vi "UNIX_date.vi"(8 "error in (no error)":errorcluster) -> (0 "error out":errorcluster, 3 "current time":timestamp)   [LabVIEW 2014]
doc: "Outputs the current UNIX time (converts from the 1904 epoch LabVIEW based time to the 1970 UNIX epoch time). In addition, this VI takes into account the current time zone (and daylight saving settings) you have on your computer to get the accurate UNIX time conversion."
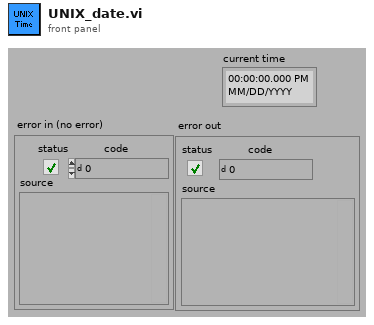
[diagram p1: front panel]
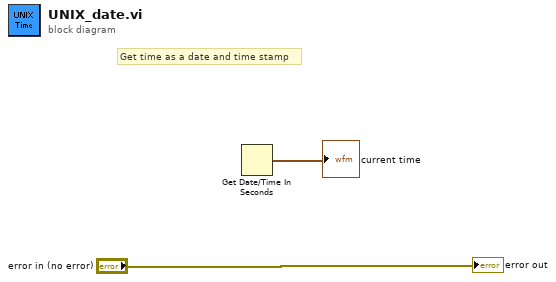
[diagram p0: block diagram]
diagram:
  # "Get time as a date and time stamp"
  n1 = Get Date/Time In Seconds() -> (seconds since 1Jan1904=→"current time":timestamp)
  "error out" <- "error in (no error)"
